vi "Set package_template_enum.vi"(7 "Complete Call (T)":bool=TRUE, 8 "error in (no error)":errorcluster, 10 "package_template_enum":T1, 11 "gRPCid":T2) -> (0 "error out":errorcluster)   [LabVIEW 2024, in "Service Template.lvlib"]
uses:
  Service Template.lvlib
  gRPC lv Support/grpc-lvsupport/grpcId.ctl
  package_templatemessage.ctl
  dcc74a39-081a-4bdd-860b-8ed792803c96.vi
  gRPC lv Support/grpc-lvsupport/TranslateGrpcError.vi
  <vilib>/Utility/error.llb/Error Cluster From Error Code.vi
  gRPC lv Support/grpc-lvsupport/grpc-lvsupport.lvlib
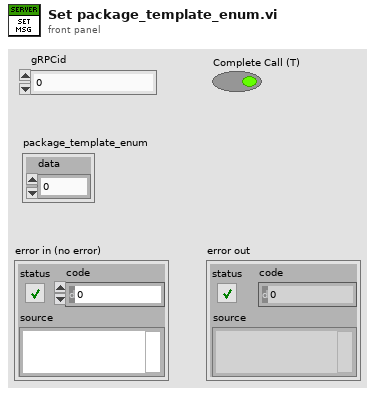
[diagram p1: front panel]
types:
  T1 = typedef "Service Template.lvlib/package_templatemessage.ctl" = cluster{"data":sgl}
  T2 = typedef "grpc-lvsupport.lvlib/grpcId.ctl" = u64
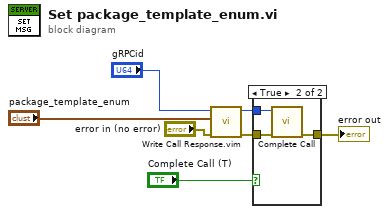
[diagram p0: block diagram]
diagram:
  n1 = call "Write Call Response.vim"("error in"="error in (no error)", "Response Data"="package_template_enum", "gRPCid in"="gRPCid") -> ("error out"=w4:errorcluster, "gRPCid out"=w5:T2)  [unwired: 7 in]
  n2 = case shown="True" "Complete Call (T)" {
    tunnel: [w8 w11] -> w7
    tunnel: w5 -> [_ w10]
    tunnel: w4 -> [w8 w9]
    frame False {
    }
    frame True {
      n3 = call "Complete Call.vi"("gRPCid"=w10, "error in"=w9) -> ("error out"=w11:errorcluster)  [unwired: 8 in]
    }
  }
  "error out" <- w7
